vi "AAA Emrax 228 Testing.vi"() -> ()   [LabVIEW 2020]
uses:
  <instrlib>/Gantner Instruments/Ethernet/Gantner-Instruments HighSpeedPort.llb/e.gate Protocol Type.ctl
  <vilib>/Instr/_visa.llb/VISA Configure Serial Port (Instr).vi
  <vilib>/Utility/file.llb/Write Delimited Spreadsheet (string).vi
panel:
  out "Value":dbl[](graph)
  out "Brake pot Input":u32
  out "Torque Shudder":u32
  out "Motor Temp":u32(slide) scale=0.0..100.0
  out "Inverter Temp":u32(slide) scale=0.0..100.0
  out "Modulation":u32
  in  "string":string
  out "error out 3":errorcluster
  out "Motor Voltage Magnitude":u32
  out "Flux weakening regulator":u32
  out "RPM Feedback":u32(knob) scale=0.0..6000.0
  out "?":u32(knob) scale=0.0..60.0
  out "?":u32(knob) scale=0.0..60.0
  out "Torque Command":u32
  out "Torque Feedback":u32
  out "Potmeter Input":u32
  out "Elapsed Time":u32
  out "return count":u32
  out "Humidity (%)":string
  out "Pressure (Pa)":string
  out "Temperature (°C)":string
  out "Elapsed Time":string
  out "?":dbl[](array[slide]) scale=0.0..1000.0
  out "Temperature 2":dbl[](array[slide]) caption="Thermocouple 1" scale=20.0..50.0
  out "error out 2":errorcluster
  in  "?":bool
  out "error out":errorcluster
  # "Emrax 228  -  Motor control"
  # "Battery Data"
  # "Temperatures"
  # "Torque"
  # "Power Supply"
  # "DC Voltage"
  # "Atmospheric\nConditions"
  # "Thrust"
  # "DC Current"
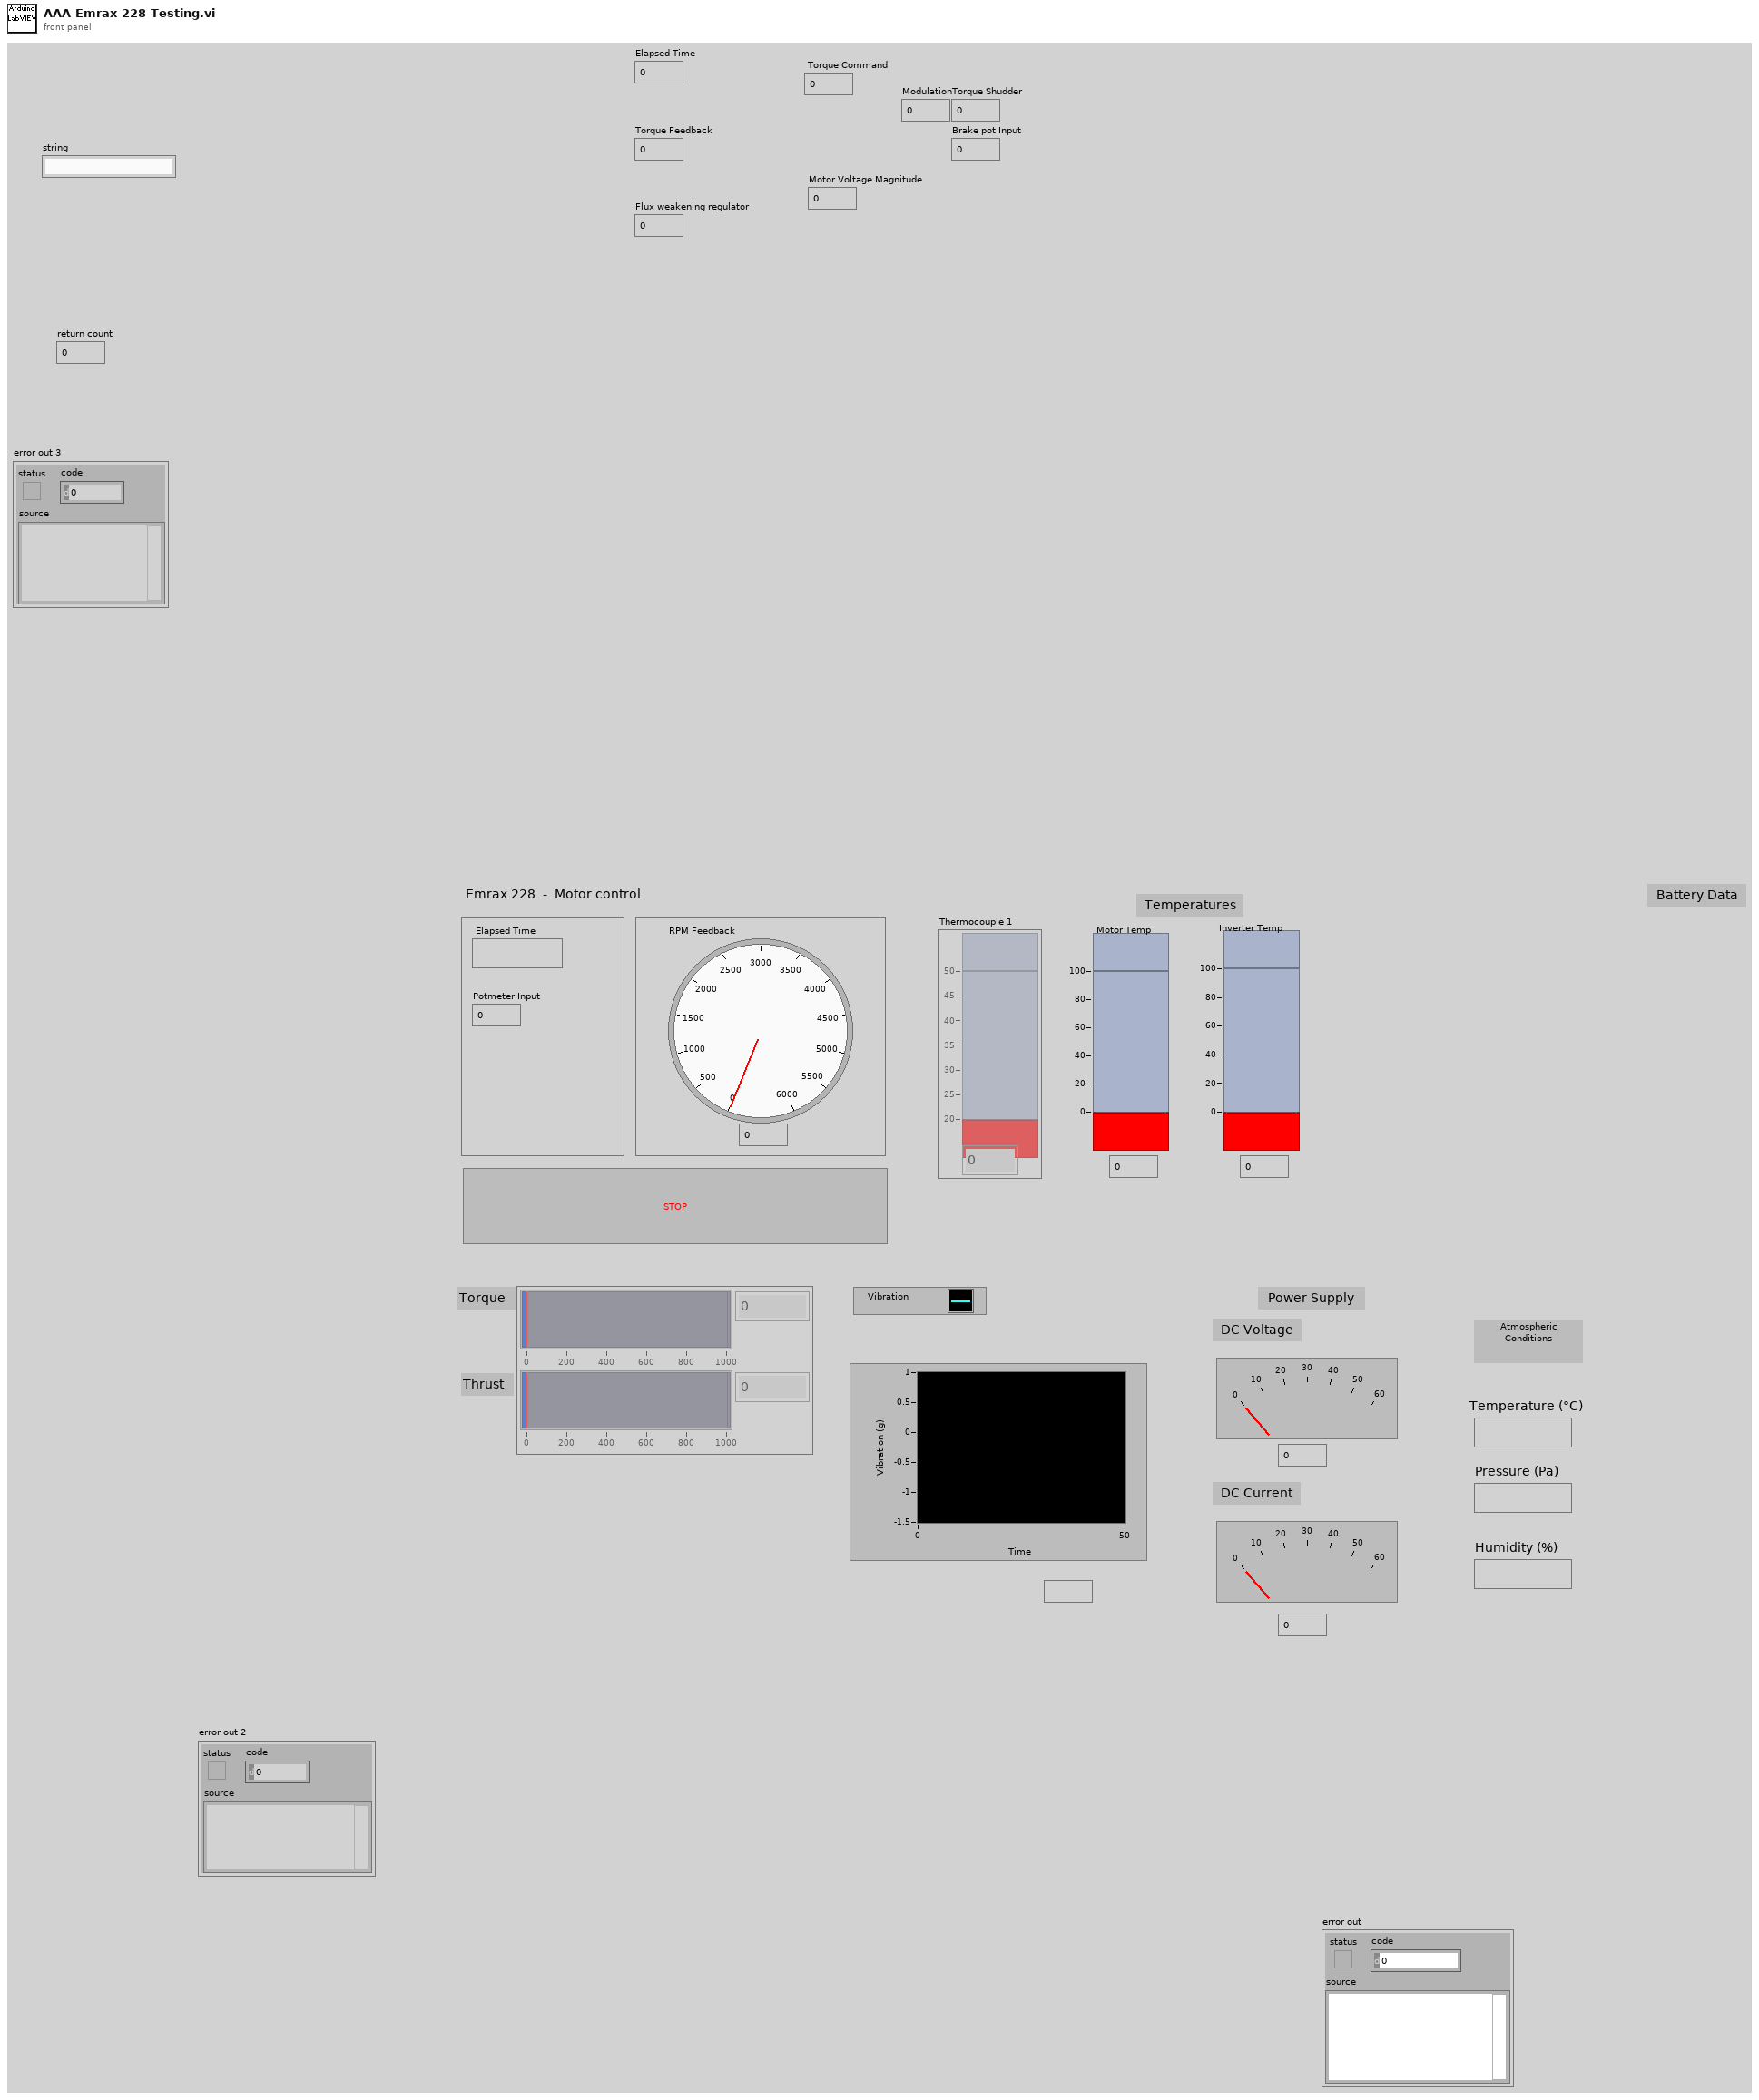
[diagram p1: front panel]
types:
  T1 = typedef "e.gate Protocol Type.ctl" = enum16{"ASCII", "HighspeedPort Online", "HighspeedPort Buffer (giutility.DLL) ", "PostProcessBuffer (giutility.DLL)", "HighspeedPort Online (giutility.DLL)", "Decode UDBF File (giutility.DLL)"}
  T2 = typedef "e.gate Configuration.ctl" = cluster{"connection ID":refnum<k5>, "IPAddress":string, "BufferIndex":i32, "StateMessage":string, "StateCode":i8, "HeaderSize":i32, "BufferSize":i32, "IsBigEndian":i32, "Version":i32, "ChannelCount":i32, "FrameLength":i32, "StartTime":dbl, "dActTimeToSecondFactor":dbl, "StartTimeToDayFactor":dbl, "BufferFillRate":dbl, "SampleRate":dbl, "ChannelData":T3[], "DecodeTimeFormat":string, "SummaryPath":string, "WithCheckSum":i32, "dActTimeDataType":T4, "MaxWriteCount":i32, "MaxReadCount":i32, "TempOffsetRead":i32, "TempLengthRead":i32, "Protocol":T1, "IsSupported":i32, "InputAccessList":i32[], "OutputAccessList":i32[], "DataSource":enum16{"CircleBuffer", "test.con Logger", "test.con Archive"}, "Modules":T5[], "DLL-Handle":T6}
  T3 = typedef "e.gate Channel Data.ctl" = cluster{"VariableName":string, "DataDirection":string, "DataType":string, "DataTypeIndex":T4, "Precision":i16, "FieldLengtht":i16, "ByteCount":i32, "Format":string, "Unit":string, "InputAccessOffset":i32, "OutputAccessOffset":i16, "InputAccessIndex":i16, "OutputAccessIndex":i16, "VarType":string}
  T4 = typedef "e.gate Data Type.ctl" = enum16{"NO", "BOOL", "SINT8", "USINT8", "SINT16", "USINT16", "SINT32", "USINT32", "FLOAT", "SET8", "SET16", "SET32", "DOUBLE", "SINT64", "USINT64", "SET64"}
  T5 = typedef "e.gate Module  Data.ctl" = cluster{"Type":string, "Location":string, "VariablesCount":i16, "UartIndex":i16, "Address":i16, "SystemOffset":i16}
  T6 = typedef "e.gateHSP_DLLhandle.ctl" = cluster{"clientInstance":i32, "connectionInstance":i32, "Is32Bit":bool, "DLL Path":path}
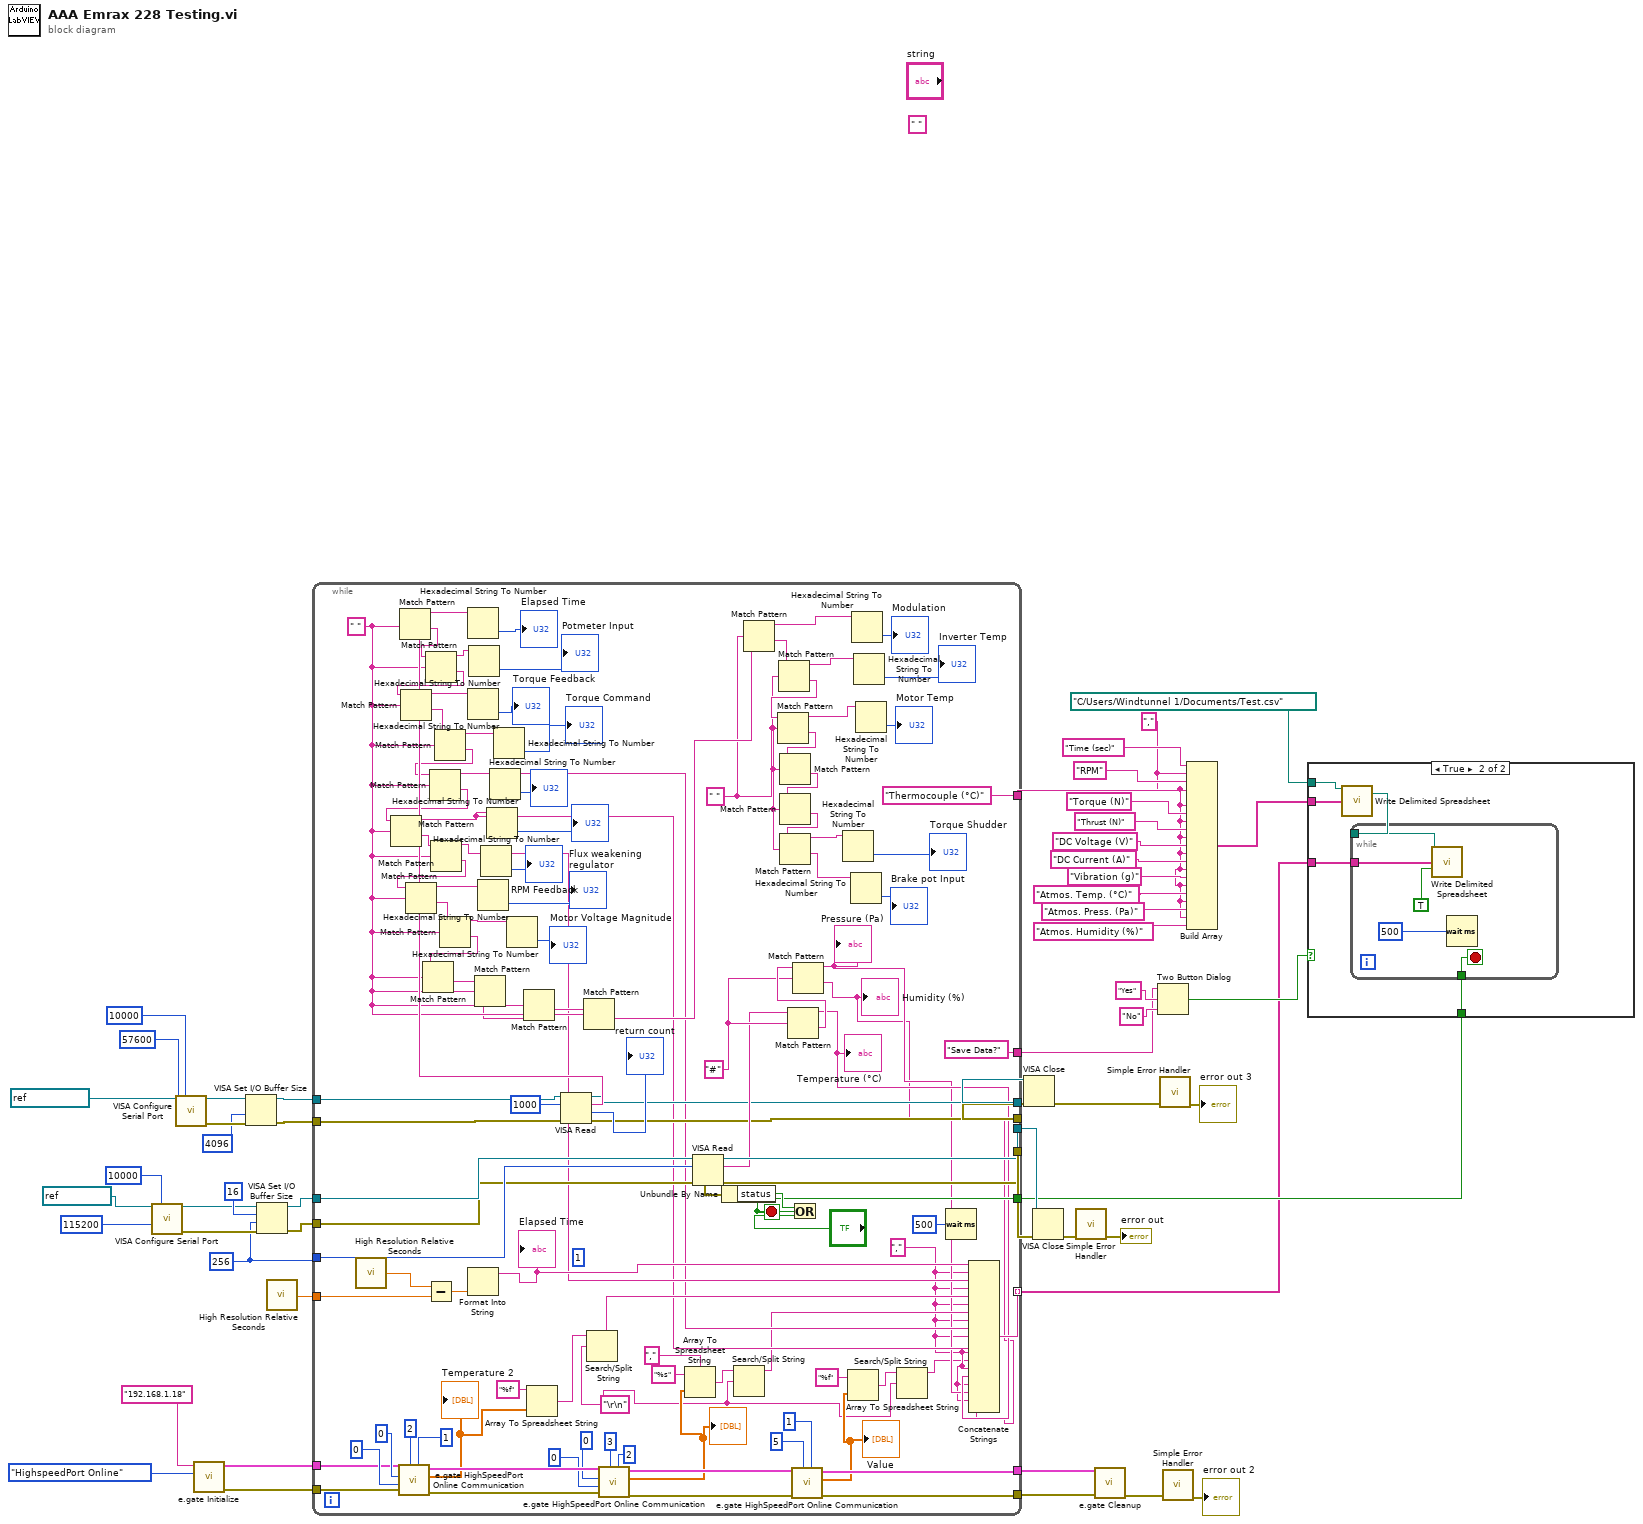
[diagram p0: block diagram]
diagram:
  (unwired) " " ("search string/char (-)")
  w2 = "," ("element")
  w42 = u32 256 ("buffer size")
  n1 = call-poly "VISA Configure Serial Port"("VISA resource name"=refnum<visa-resource-name> "COM5", "timeout (10sec)"=u32 10000, "baud rate (9600)"=u32 115200) -> ("VISA resource name out"=w51:refnum<visa-resource-name>, "error out"=w50:errorcluster)  [unwired: 11 in]
  n2 = call-poly "VISA Configure Serial Port"("VISA resource name"=refnum<visa-resource-name> "COM6", "timeout (10sec)"=u32 10000, "baud rate (9600)"=u32 57600) -> ("VISA resource name out"=w19:refnum<visa-resource-name>, "error out"=w18:errorcluster)  [unwired: 11 in]
  n3 = call <instrlib>:"e.gate Initialize.vi"("Protocol"=e.gate_Protocol_Type."HighspeedPort Online", "IP Address"="192.168.1.18") -> ("error out"=w36:errorcluster, "e.gate Configuration"=w37:T2)  [unwired: 8 in]
  n4 = VISA Set I/O Buffer Size(VISA resource name=w19, size (4096)=u32 4096, error in (no error)=w18) -> (VISA resource name out=w13:refnum<visa-resource-name>, error out=w12:errorcluster)  [unwired: 1 in]
  n5 = VISA Set I/O Buffer Size(VISA resource name=w51, mask (16)=u16 16 ("I/O Receive\nBuffer mask"), size (4096)=w42, error in (no error)=w50) -> (VISA resource name out=w49:refnum<visa-resource-name>, error out=w48:errorcluster)
  n6 = call <vilib>:"High Resolution Relative Seconds.vi"() -> ("relative seconds"=w27:dbl)
  n7 = while {
    tunnel: w49 -> [w134]
    tunnel: w48 -> [w133]
    tunnel: [w163] -> w54
    tunnel: [w161] -> w53
    tunnel: w42 -> [w164]
    tunnel: w37 -> [w148]
    tunnel: w36 -> [w147]
    tunnel: [w77] -> w35
    tunnel: [w75] -> w34
    tunnel: [w146] -> w29
    tunnel: w27 -> [w143]
    tunnel: [w67] -> w28 mode=indexing
    tunnel: w13 -> [w105]
    tunnel: w12 -> [w104]
    tunnel: [w103] -> w11
    tunnel: [w102] -> w10
    tunnel: ["Thermocouple (°C)" ("element")] -> w9
    tunnel: ["Save Data?" ("message")] -> w8
    stop <- w146 stop-if-true
    w56 = "\r\n" ("search string/char (-)")
    w89 = " " ("search string/char (-)")
    w99 = " " ("search string/char (-)")
    w135 = "#" ("regular expression")
    (unwired) 1 ("offset (0)")
    w59 = "," ("string")
    n8 = call <vilib>:"High Resolution Relative Seconds.vi"() -> ("relative seconds"=w144:dbl)
    n9 = call <instrlib>:"e.gate HighSpeedPort Online Communication.vi"("ReadCount"=1, "ReadIndex"=2, "error in (no error)"=w147, "WriteCount"=0, "WriteIndex"=0, "e.gate Configuration In"=w148) -> ("error out"=w153:errorcluster, "Value"=w145:dbl[], "e.gate Configuration Out"=w154:T2)  [unwired: 3 in]
    "Temperature 2" <- w145
    n10 = Subtract(x=w144, y=w143) -> (x-y=w142:dbl)
    n11 = Format Into String(w142) -> (resulting string=w71:string)  [unwired: 3 in, 1 out]
    "Elapsed Time" <- w71
    n12 = Array To Spreadsheet String(array=w145, 3:"%f" ("format string")) -> (spreadsheet string=w138:string)  [unwired: 1 in]
    n13 = VISA Read(VISA resource name=w105, byte count=u32 1000, error in (no error)=w104) -> (VISA resource name out=w103:refnum<visa-resource-name>, read buffer=w122:string, return count=→"return count":u32, error out=w102:errorcluster)
    n14 = Match Pattern(string=w122, regular expression=w99) -> (before substring=w108:string, after substring=w110:string)  [unwired: 1 in, 2 out]
    n15 = Match Pattern(string=w110, regular expression=w99) -> (before substring=w111:string, after substring=w113:string)  [unwired: 1 in, 2 out]
    n16 = Match Pattern(string=w113, regular expression=w99) -> (before substring=w114:string, after substring=w116:string)  [unwired: 1 in, 2 out]
    n17 = Match Pattern(string=w116, regular expression=w99) -> (before substring=w117:string, after substring=w119:string)  [unwired: 1 in, 2 out]
    n18 = Match Pattern(string=w119, regular expression=w99) -> (before substring=w65:string, after substring=w121:string)  [unwired: 1 in, 2 out]
    n19 = Match Pattern(string=w121, regular expression=w99) -> (before substring=w64:string, after substring=w124:string)  [unwired: 1 in, 2 out]
    n20 = Match Pattern(string=w124, regular expression=w99) -> (before substring=w70:string, after substring=w126:string)  [unwired: 1 in, 2 out]
    n21 = Match Pattern(string=w126, regular expression=w99) -> (before substring=w127:string, after substring=w129:string)  [unwired: 1 in, 2 out]
    n22 = Match Pattern(string=w129, regular expression=w99) -> (before substring=w130:string, after substring=w100:string)  [unwired: 1 in, 2 out]
    n23 = Match Pattern(string=w100, regular expression=w99) -> (after substring=w98:string)  [unwired: 1 in, 3 out]
    n24 = Hexadecimal String To Number(string=w108) -> (number=→"Elapsed Time":u32)  [unwired: 2 in, 1 out]
    n25 = Hexadecimal String To Number(string=w114) -> (number=→"Torque Feedback":u32)  [unwired: 2 in, 1 out]
    n26 = Hexadecimal String To Number(string=w111) -> (number=→"Potmeter Input":u32)  [unwired: 2 in, 1 out]
    n27 = Match Pattern(string=w98, regular expression=w99) -> (after substring=w97:string)  [unwired: 1 in, 3 out]
    n28 = Hexadecimal String To Number(string=w127) -> (number=→"Flux weakening regulator":u32)  [unwired: 2 in, 1 out]
    n29 = Hexadecimal String To Number(string=w70) -> (number=→"RPM Feedback":u32)  [unwired: 2 in, 1 out]
    n30 = Hexadecimal String To Number(string=w64) -> (number=→"?":u32)  [unwired: 2 in, 1 out]
    n31 = Hexadecimal String To Number(string=w65) -> (number=→"?":u32)  [unwired: 2 in, 1 out]
    n32 = Hexadecimal String To Number(string=w117) -> (number=→"Torque Command":u32)  [unwired: 2 in, 1 out]
    n33 = Hexadecimal String To Number(string=w130) -> (number=→"Motor Voltage Magnitude":u32)  [unwired: 2 in, 1 out]
    n34 = Match Pattern(string=w97, regular expression=w99) -> (after substring=w96:string)  [unwired: 1 in, 3 out]
    n35 = Match Pattern(string=w96, regular expression=w99) -> (after substring=w95:string)  [unwired: 1 in, 3 out]
    n36 = Search/Split String(string=w138, search string/char (-)=w56) -> (substring before match=w137:string)  [unwired: 1 in, 2 out]
    n37 = call <instrlib>:"e.gate HighSpeedPort Online Communication.vi"("ReadCount"=2, "ReadIndex"=3, "error in (no error)"=w153, "WriteCount"=0, "WriteIndex"=0, "e.gate Configuration In"=w154) -> ("error out"=w76:errorcluster, "Value"=w72:dbl[], "e.gate Configuration Out"=w78:T2)  [unwired: 3 in]
    "?" <- w72
    n38 = Array To Spreadsheet String(delimiter (Tab)=",", array=w72, 3:"%s" ("format string")) -> (spreadsheet string=w63:string)
    n39 = VISA Read(VISA resource name=w134, byte count=w164, error in (no error)=w133) -> (VISA resource name out=w163:refnum<visa-resource-name>, read buffer=w132:string, error out=w161:errorcluster)  [unwired: 1 out]
    n40 = Unbundle By Name(w161) -> ("status"=w160:bool)
    n41 = Search/Split String(string=w63, search string/char (-)=w56) -> (substring before match=w62:string)  [unwired: 1 in, 2 out]
    n42 = Match Pattern(string=w95, regular expression=w89) -> (before substring=w88:string, after substring=w94:string)  [unwired: 1 in, 2 out]
    n43 = Match Pattern(string=w94, regular expression=w89) -> (before substring=w87:string, after substring=w93:string)  [unwired: 1 in, 2 out]
    n44 = Match Pattern(string=w93, regular expression=w89) -> (before substring=w86:string, after substring=w92:string)  [unwired: 1 in, 2 out]
    n45 = Match Pattern(string=w92, regular expression=w89) -> (after substring=w91:string)  [unwired: 1 in, 3 out]
    n46 = Match Pattern(string=w91, regular expression=w89) -> (after substring=w90:string)  [unwired: 1 in, 3 out]
    n47 = Match Pattern(string=w90, regular expression=w89) -> (before substring=w85:string, after substring=w79:string)  [unwired: 1 in, 2 out]
    n48 = Match Pattern(string=w132, regular expression=w135) -> (before substring=w61:string, after substring=w136:string)  [unwired: 1 in, 2 out]
    "Temperature (°C)" <- w61
    n49 = Or(x=w160, y="?") -> (x .or. y?=w146:bool)
    n50 = call <instrlib>:"e.gate HighSpeedPort Online Communication.vi"("ReadCount"=1, "ReadIndex"=5, "error in (no error)"=w76, "e.gate Configuration In"=w78) -> ("error out"=w75:errorcluster, "Value"=w69:dbl[], "e.gate Configuration Out"=w77:T2)  [unwired: 5 in]
    "Value" <- w69
    n51 = Match Pattern(string=w136, regular expression=w135) -> (before substring=w60:string, after substring=w58:string)  [unwired: 1 in, 2 out]
    "Pressure (Pa)" <- w60
    "Humidity (%)" <- w58
    n52 = Hexadecimal String To Number(string=w85) -> (number=→"Torque Shudder":u32)  [unwired: 2 in, 1 out]
    n53 = Array To Spreadsheet String(array=w69, 3:"%f" ("format string")) -> (spreadsheet string=w57:string)  [unwired: 1 in]
    n54 = Hexadecimal String To Number(string=w79) -> (number=→"Brake pot Input":u32)  [unwired: 2 in, 1 out]
    n55 = Hexadecimal String To Number(string=w88) -> (number=→"Modulation":u32)  [unwired: 2 in, 1 out]
    n56 = Hexadecimal String To Number(string=w87) -> (number=→"Inverter Temp":u32)  [unwired: 2 in, 1 out]
    n57 = Hexadecimal String To Number(string=w86) -> (number=→"Motor Temp":u32)  [unwired: 2 in, 1 out]
    n58 = Search/Split String(string=w57, search string/char (-)=w56) -> (substring before match=w55:string)  [unwired: 1 in, 2 out]
    n59 = Wait (ms)(milliseconds to wait=u32 500) -> ()  [unwired: 1 out]
    n60 = Concatenate Strings(w71, w59, w70, w59, w137, w59, w62, w59, w65, w59, w64, w59, w55, w59, w61, w59, w60, w59, w58) -> (w67:string)
  }
  n61 = VISA Close(VISA resource name=w11, error in (no error)=w10) -> (error out=w21:errorcluster)
  n62 = VISA Close(VISA resource name=w54, error in (no error)=w53) -> (error out=w47:errorcluster)
  n63 = call <vilib>:"Simple Error Handler.vi"("error in (no error)"=w47) -> ("error out"=→"error out":errorcluster)  [unwired: 4 in, 4 out]
  n64 = call <instrlib>:"e.gate Cleanup.vi"("error in (no error)"=w34, "e.gate Configuration"=w35) -> ("error out"=w41:errorcluster)  [unwired: 9 in]
  n65 = Two Button Dialog(message=w8, 1:"No" ("F button name (\"Cancel\")"), 2:"Yes" ("T button name (\"OK\")")) -> (T button?=w32:bool)
  n66 = call <vilib>:"Simple Error Handler.vi"("error in (no error)"=w21) -> ("error out"=→"error out 3":errorcluster)  [unwired: 4 in, 4 out]
  n67 = call <vilib>:"Simple Error Handler.vi"("error in (no error)"=w41) -> ("error out"=→"error out 2":errorcluster)  [unwired: 4 in, 4 out]
  n68 = Build Array("Time (sec)" ("element"), w2, "RPM" ("element"), w2, w9, w2, "Torque (N)" ("element"), w2, "Thrust (N)" ("element"), w2, "DC Voltage (V)" ("element"), w2, "DC Current (A)" ("element"), w2, "Vibration (g)" ("element"), w2, "Atmos. Temp. (°C)" ("element"), w2, "Atmos. Press. (Pa)" ("element"), w2, "Atmos. Humidity (%)" ("element")) -> (w33:string[])
  n69 = case shown="True" w32 {
    tunnel: w33 -> [_ w168]
    tunnel: w29 -> [_ w167]
    tunnel: w28 -> [_ w166]
    tunnel: path "C:/Users/Windtunnel 1/Documents/Test.csv" ("file path (dialog if empty) 2") -> [_ w165]
    frame False {
    }
    frame True {
      n70 = call-poly <vilib>:"Write Delimited Spreadsheet.vi"("file path (dialog if empty)"=w165, "1D data"=w168) -> ("new file path (Not A Path if cancelled)"=w169:path)  [unwired: 12 in, 1 out]
      n71 = while {
        tunnel: w169 -> [w174]
        tunnel: w167 -> [w171]
        tunnel: w166 -> [w170]
        stop <- w171 stop-if-true
        n72 = call-poly <vilib>:"Write Delimited Spreadsheet.vi"("file path (dialog if empty)"=w174, "1D data"=w170, "append to file? (new file:F)"=TRUE) -> ()  [unwired: 11 in, 2 out]
        n73 = Wait (ms)(milliseconds to wait=u32 500) -> ()  [unwired: 1 out]
      }
    }
  }
